vi "setpoint_computation.vi"(1 "activate":bool, 2 "Req":dbl, 3 "Meas":dbl) -> (0 "SP":dbl)   [LabVIEW 2021]
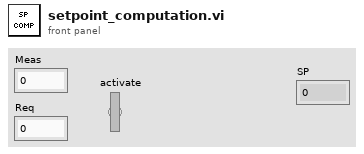
[diagram p1: front panel]
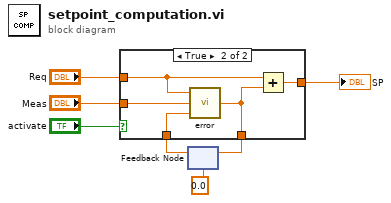
[diagram p0: block diagram]
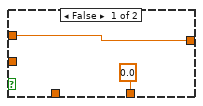
[diagram p2: hidden frame]
diagram:
  n1 = feedback #1(0.0 ("error (out)")) -> (w1:dbl)
  n2 = case shown="True" "activate" {
    tunnel: [w9 w14] -> w6
    tunnel: "Req" -> [w9 w13]
    tunnel: "Meas" -> [_ w12]
    tunnel: [0.0 ("error (out)") w11] -> w2
    tunnel: w1 -> [_ w10]
    frame False {
    }
    frame True {
      n3 = call "error.vi"("error (in)"=w10, "Meas"=w12, "Req"=w13) -> ("error (out)"=w11:dbl)
      n4 = Add(x=w13, y=w11) -> (x+y=w14:dbl)
    }
  }
  "SP" <- w6
  n5 = feedback-in #1(w2) -> ()
